vi "Frames.Initialize.vi"(8 "error in":errorcluster, 9 "Lookup":variant, 10 "Frames":T1[](array[typedef]) {"Signals"."Byte Order" items=["Little Endian", "Big Endian"]; "Signals"."Data Type" items=["Signed", "Unsigned", "IEEE Float"]}, 11 "Cluster In":refnum<k21>) -> (0 "error out":errorcluster, 1 "Lookup":variant, 3 "Cluster Out":refnum<k21>)   [LabVIEW 2019, in "Diagnostics Addon Engine.lvlib"]
uses:
  Diagnostics Addon Engine.lvlib
  Shared/Types/Frame.Compile.ctl
  Shared/Types/Type.ctl
  Shared/Types/Signal.ctl
  Shared/Types/XNET.Frame.ctl
  Shared/SubVIs/Constants.vi
  <vilib>/xnet/xnet.llb/XNET Create Session (Conversion).vi
  Shared/Diagnostics Addon Shared.lvlib
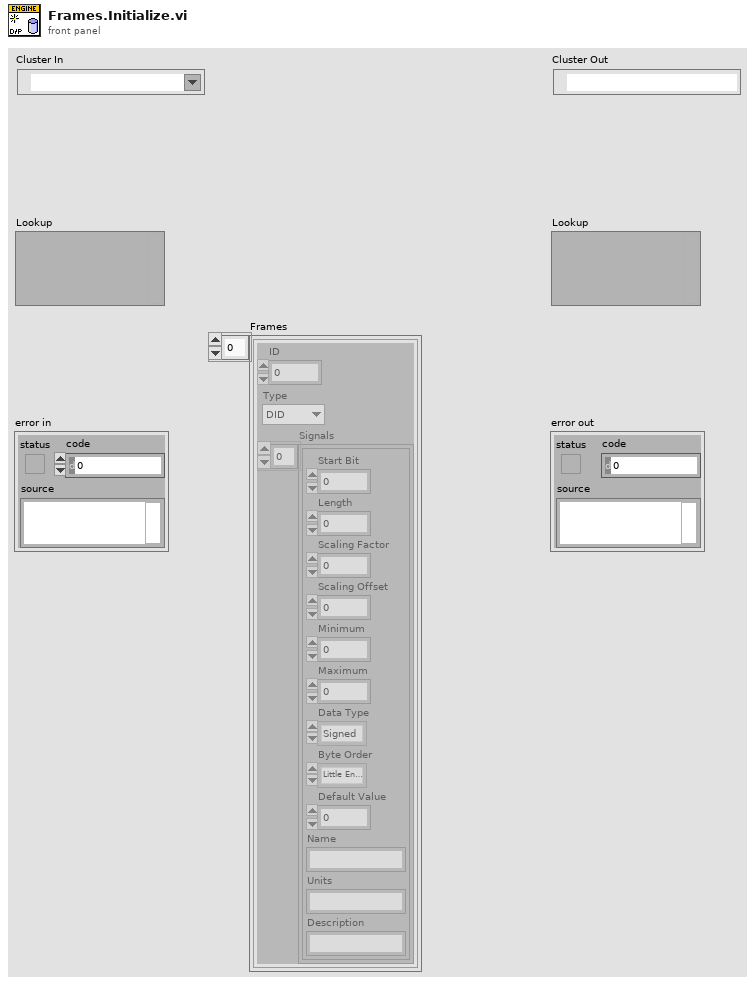
[diagram p1: front panel]
types:
  T1 = typedef "Diagnostics Addon Shared.lvlib/Frame.Compile.ctl" = cluster{"ID":u32, "Type":T2, "Signals":T3[]}
  T2 = typedef "Diagnostics Addon Shared.lvlib/Type.ctl" = enum16{"DID", "CDID", "PID", "CPID", "Read Memory", "Write Memory", "DTC Control", "IO Cmd", "IO Resp", "Routine Start Cmd", "Routine Start Resp", "Routine Request Cmd", "Routine Request Resp", "Routine Stop Cmd", "Routine Stop Resp", "UserDefined Cmd", "UserDefined Rsp"}
  T3 = typedef "Diagnostics Addon Shared.lvlib/Signal.ctl" = cluster{"Start Bit":u32, "Length":u32, "Scaling Factor":dbl, "Scaling Offset":dbl, "Minimum":dbl, "Maximum":dbl, "Data Type":u32, "Byte Order":u32, "Default Value":dbl, "Name":string, "Units":string, "Description":string}
  T4 = typedef "Diagnostics Addon Shared.lvlib/XNET.Frame.ctl" = cluster{"Frame name":string, "Identifier":u32, "Payload Length":u32, "Timing Type":u32, "Transmit Time":dbl, "Extended Identifier?":bool, "Comment":string}
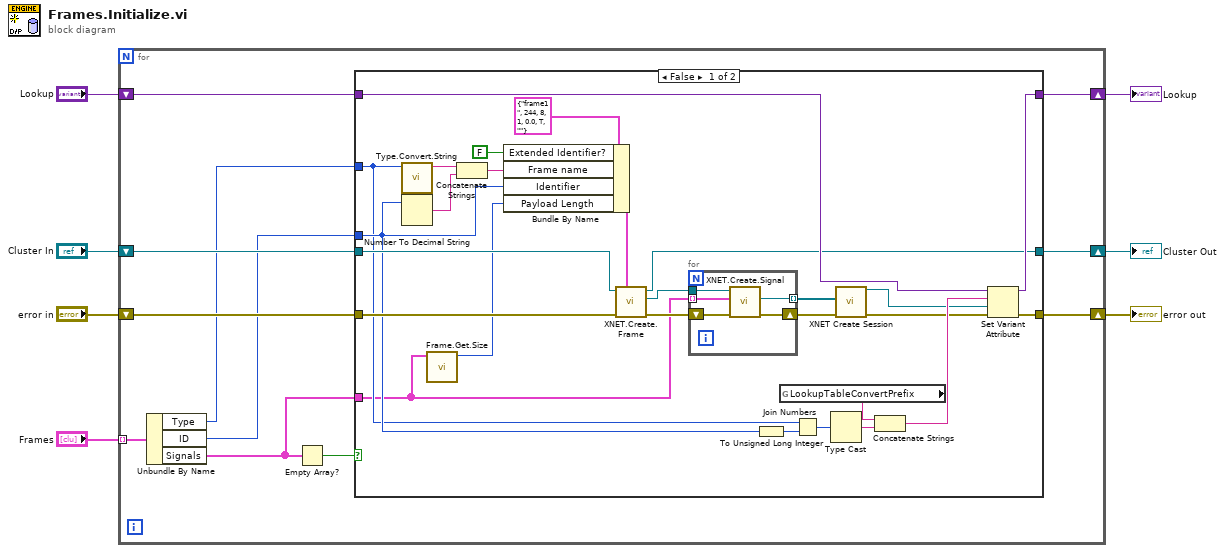
[diagram p0: block diagram]
diagram:
  n1 = for {
    shift-right: [w17] -> w6
    shift-left: "error in" -> [w14]
    tunnel: "Frames" -> [w18] mode=indexing
    shift-right: [w15] -> w4
    shift-left: "Lookup" -> [w16]
    shift-right: [w12] -> w1
    shift-left: "Cluster In" -> [w13]
    n2 = Unbundle By Name(w18) -> ("Type"=w10:T2, "ID"=w11:u32, "Signals"=w9:T3[])
    n3 = Empty Array?(array=w9) -> (empty?=w8:bool)
    n4 = case shown="False" w8 {
      tunnel: [w45 w53] -> w17
      tunnel: w16 -> [w44 w51]
      tunnel: [w43 w51] -> w15
      tunnel: w14 -> [w41 w53]
      tunnel: w13 -> [w35 w52]
      tunnel: [w33 w52] -> w12
      tunnel: w11 -> [w31 _]
      tunnel: w10 -> [w30 _]
      tunnel: w9 -> [w21 _]
      frame False {
        n5 = call "Type.Convert.String.vi"("Type"=w30) -> ("signal name"=w39:string)  [unwired: 10 in]
        n6 = Number To Decimal String(number=w31) -> (decimal integer string=w32:string)  [unwired: 1 in]
        n7 = call "Frame.Get.Size.vi"("Parameters"=w21) -> ("Bytes"=w20:u32)  [unwired: 10 in]
        n8 = Concatenate Strings(w39, w32) -> (w38:string)
        n9 = Bundle By Name(cluster=T4 {"Frame name"="frame1", "Identifier"=244, "Payload Length"=8, "Timing Type"=1, "Transmit Time"=0.0, "Extended Identifier?"=TRUE, "Comment"=""} ("CAN Frame"), "Extended Identifier?"=FALSE, "Frame name"=w38, "Identifier"=w31, "Payload Length"=w20) -> (w36:T4)
        n10 = call "XNET.Create.Frame.vi"("error in"=w41, "CAN Frame"=w36, "cluster in"=w35) -> ("error out"=w40:errorcluster, "frame out"=w34:refnum<k21>, "cluster out"=w33:refnum<k21>)  [unwired: 6 in]
        n11 = for {
          tunnel: w34 -> [w46]
          tunnel: w21 -> [w47] mode=indexing
          shift-right: [w49] -> w42
          shift-left: w40 -> [w50]
          tunnel: [w48] -> w29 mode=indexing
          n12 = call "XNET.Create.Signal.vi"("error in"=w50, "Signal"=w47, "frame in"=w46) -> ("error out"=w49:errorcluster, "signal out"=w48:refnum<k21>)  [unwired: 6 in, 1 out]
        }
        n13 = To Unsigned Long Integer(number=w31) -> (unsigned 32bit integer=w23:u32)
        n14 = global read "Constants.vi" "LookupTableConvertPrefix"() -> (w28:string)
        n15 = Join Numbers(hi=w30, lo=w23) -> ((hi.lo)=w22:u64)
        n16 = Type Cast(x=w22) -> (*(type *) &x=w24:string)  [unwired: 1 in]
        n17 = call-poly <vilib>:"XNET Create Session.vi"("signal list"=w29, "error in (no error)"=w42) -> ("session out"=w25:refnum<k21>, "error out"=w26:errorcluster)  [unwired: 1 in, 11 out]
        n18 = Concatenate Strings(w28, w24) -> (w27:string)
        n19 = Set Variant Attribute(Variant=w44, name=w27, value=w25, error in=w26) -> (Variant out=w43:variant, error out=w45:errorcluster)  [unwired: 1 out]
      }
      frame True {
      }
    }
  }
  "error out" <- w6
  "Cluster Out" <- w1
  "Lookup" <- w4
